vi "Juicer-ChangeMode.vi"(7 "Device reference":refnum<vi>, 8 "error in (no error)":errorcluster, 9 "Eventstring":string="auto-generate", 11 "Mode":enum16{"off", "reward", "flush", "purge"}(ring)) -> (0 "error out":errorcluster)   [LabVIEW 2015]
doc: "Changes the mode of a juicer device.\n\nDevice reference: what juicer?\nMode: what mode to switch to?\n off: All disconnected\n reward: Reward tank connected\n flush: Water flush tank connected\n purge: Pressurized air connected\nEventstring: used for timestamping\n--empty: no timestamp will be generated\n--unwired or \"auto-generate\": TS w/ default eventstring\n--otherwise: TS with user-provided string\n\nThe default eventstring is:\n[juicer name].changeMode.[mode]\n\nThis action involves multiple digital output writes; only the last one is timestamped."
uses:
  Typedefs/Juicer.ctl
  Rack/Typedefs/OutputRequest refnum.ctl
  Rack/Typedefs/OutputRequest.ctl
  Rack/Typedefs/InputData cluster.ctl
  Rack/Methods/Port drivers/DigitalInput-DataCluster.ctl
panel:
  # "(must be on same NI card)"
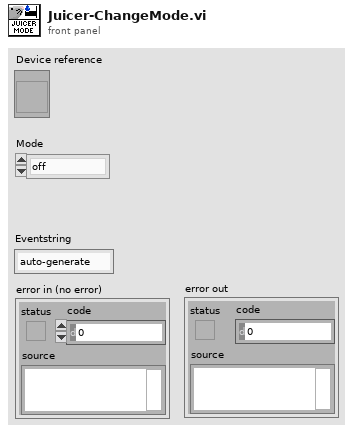
[diagram p1: front panel]
types:
  T1 = typedef "Juicer.ctl" = cluster{"Mode":enum16{"Off", "Juice/reward", "Water flush", "Air purge"}, "Settings":cluster{"Bleed #1 port index":i32, "Bleed #1 port name":string, "Bleed #2 port name":string, "Bleed #2 port index":i32, "Flush port name":string, "Flush port index":i32, "Purge port name":string, "Purge port index":i32, "Timestamp port name":string}, "OutputRequest event ref":T2, "InputData reference":refnum<vi>}
  T2 = typedef "OutputRequest refnum.ctl" = refnum<user-event>
  T3 = enum16{"Off", "Juice/reward", "Water flush", "Air purge"}
  T4 = typedef "OutputRequest.ctl" = cluster{"Target":string, "Command":string}
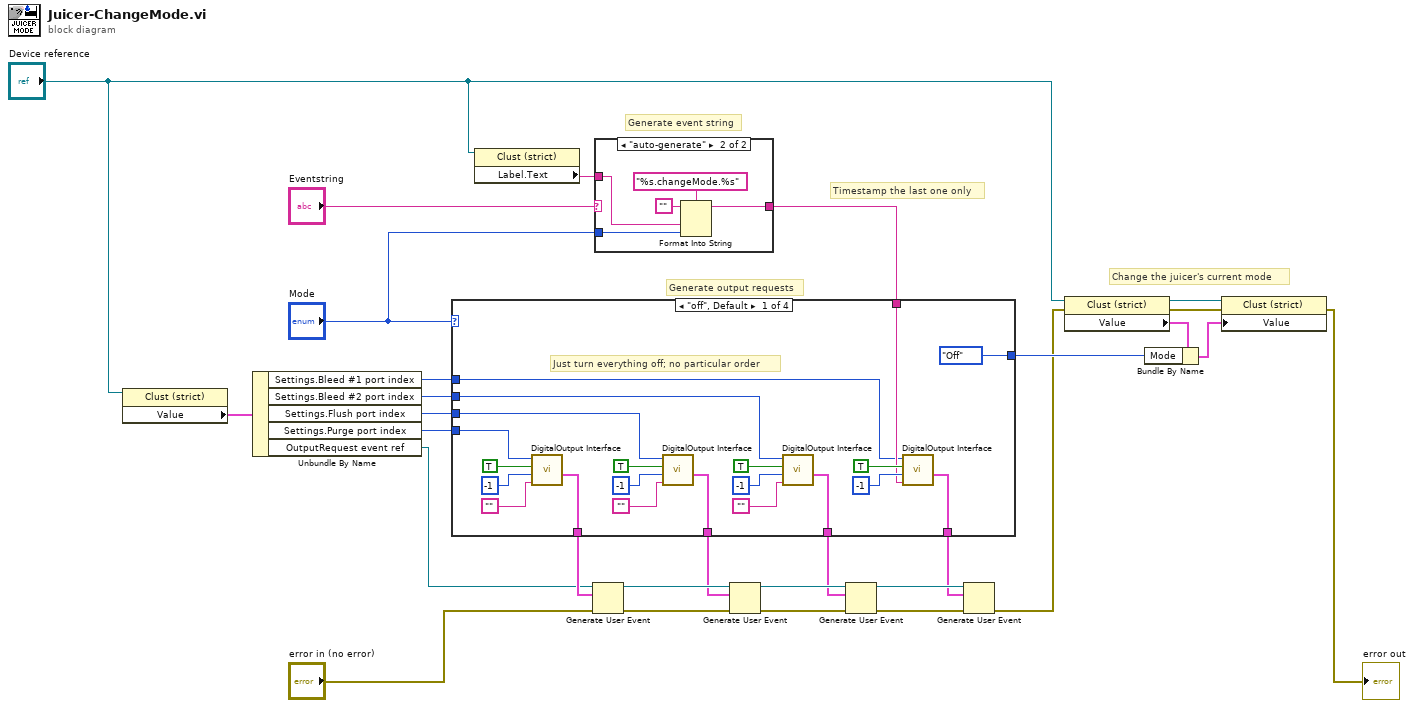
[diagram p0: block diagram]
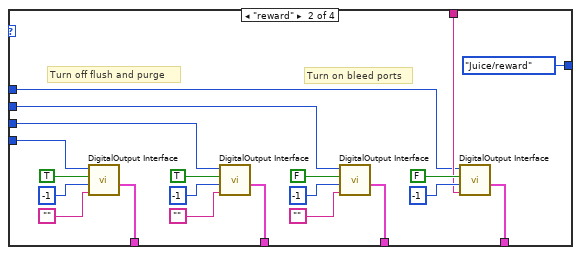
[diagram p2: hidden frame]
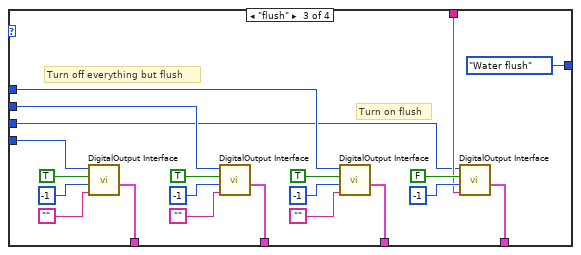
[diagram p3: hidden frame]
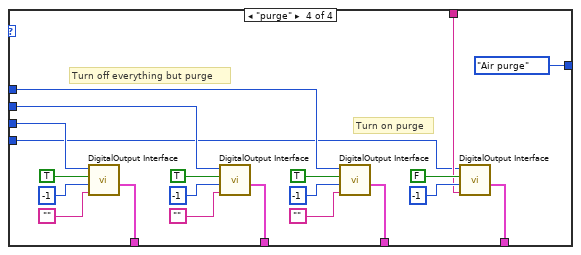
[diagram p4: hidden frame]
diagram:
  # "Change the juicer's current mode"
  # "Generate output requests"
  # "Timestamp the last one only"
  # "Generate event string"
  n1 = property class="Clust (strict)"(reference="Device reference") -> ("Value"=w29:T1)  [unwired: 1 in, 2 out]
  n2 = Unbundle By Name(w29) -> ("Settings.Bleed #1 port index"=w26:i32, "Settings.Bleed #2 port index"=w25:i32, "Settings.Flush port index"=w24:i32, "Settings.Purge port index"=w23:i32, "OutputRequest event ref"=w2:T2)
  n3 = property class="Clust (strict)"(reference="Device reference") -> ("Label.Text"=w27:string)  [unwired: 1 in, 2 out]
  n4 = case shown="\"auto-generate\"" "Eventstring" {
    selector: "Eventstring" -> [w30 _]
    tunnel: [w30 w33] -> w21
    tunnel: w27 -> [_ w32]
    tunnel: "Mode" -> [_ w31]
    frame Default {
      # "Use user-provided string"
    }
    frame "auto-generate" {
      n5 = Format Into String(format string="%s.changeMode.%s", initial string="", w32, w31) -> (resulting string=w33:string)  [unwired: 1 in, 1 out]
    }
  }
  n6 = case shown="\"off\", Default" "Mode" {
    tunnel: w26 -> [w40 w61 w80 w101]
    tunnel: w25 -> [w41 w62 w81 w102]
    tunnel: w24 -> [w42 w63 w79 w103]
    tunnel: w23 -> [w53 w74 w95 w100]
    tunnel: [w52 w73 w94 w116] -> w13
    tunnel: w21 -> [w43 w64 w85 w107]
    tunnel: [w39 w60 w84 w106] -> w12
    tunnel: [w38 w59 w83 w105] -> w11
    tunnel: [w37 w58 w82 w104] -> w10
    tunnel: [T3."Off" ("Mode") T3."Juice/reward" ("Mode") T3."Water flush" ("Mode") T3."Air purge" ("Mode")] -> w8
    frame "off", Default {
      # "Just turn everything off; no particular order"
      n7 = call "DigitalOutput Interface.vi"("Eventstring"="", "Pulse duration (-1 for cont.)"=-1, "On/off"=TRUE, "Port index"=w53) -> ("OutputRequest"=w52:T4)  [unwired: 7 in]
      n8 = call "DigitalOutput Interface.vi"("Eventstring"="", "Pulse duration (-1 for cont.)"=-1, "On/off"=TRUE, "Port index"=w42) -> ("OutputRequest"=w39:T4)  [unwired: 7 in]
      n9 = call "DigitalOutput Interface.vi"("Eventstring"="", "Pulse duration (-1 for cont.)"=-1, "On/off"=TRUE, "Port index"=w41) -> ("OutputRequest"=w38:T4)  [unwired: 7 in]
      n10 = call "DigitalOutput Interface.vi"("Eventstring"=w43, "Pulse duration (-1 for cont.)"=-1, "On/off"=TRUE, "Port index"=w40) -> ("OutputRequest"=w37:T4)  [unwired: 7 in]
    }
    frame "reward" {
      # "Turn on bleed ports"
      # "Turn off flush and purge"
      n11 = call "DigitalOutput Interface.vi"("Eventstring"="", "Pulse duration (-1 for cont.)"=-1, "On/off"=TRUE, "Port index"=w74) -> ("OutputRequest"=w73:T4)  [unwired: 7 in]
      n12 = call "DigitalOutput Interface.vi"("Eventstring"="", "Pulse duration (-1 for cont.)"=-1, "On/off"=TRUE, "Port index"=w63) -> ("OutputRequest"=w60:T4)  [unwired: 7 in]
      n13 = call "DigitalOutput Interface.vi"("Eventstring"="", "Pulse duration (-1 for cont.)"=-1, "On/off"=FALSE, "Port index"=w62) -> ("OutputRequest"=w59:T4)  [unwired: 7 in]
      n14 = call "DigitalOutput Interface.vi"("Eventstring"=w64, "Pulse duration (-1 for cont.)"=-1, "On/off"=FALSE, "Port index"=w61) -> ("OutputRequest"=w58:T4)  [unwired: 7 in]
    }
    frame "flush" {
      # "Turn on flush"
      # "Turn off everything but flush"
      n15 = call "DigitalOutput Interface.vi"("Eventstring"="", "Pulse duration (-1 for cont.)"=-1, "On/off"=TRUE, "Port index"=w95) -> ("OutputRequest"=w94:T4)  [unwired: 7 in]
      n16 = call "DigitalOutput Interface.vi"("Eventstring"="", "Pulse duration (-1 for cont.)"=-1, "On/off"=TRUE, "Port index"=w81) -> ("OutputRequest"=w84:T4)  [unwired: 7 in]
      n17 = call "DigitalOutput Interface.vi"("Eventstring"="", "Pulse duration (-1 for cont.)"=-1, "On/off"=TRUE, "Port index"=w80) -> ("OutputRequest"=w83:T4)  [unwired: 7 in]
      n18 = call "DigitalOutput Interface.vi"("Eventstring"=w85, "Pulse duration (-1 for cont.)"=-1, "On/off"=FALSE, "Port index"=w79) -> ("OutputRequest"=w82:T4)  [unwired: 7 in]
    }
    frame "purge" {
      # "Turn on purge"
      # "Turn off everything but purge"
      n19 = call "DigitalOutput Interface.vi"("Eventstring"="", "Pulse duration (-1 for cont.)"=-1, "On/off"=TRUE, "Port index"=w103) -> ("OutputRequest"=w116:T4)  [unwired: 7 in]
      n20 = call "DigitalOutput Interface.vi"("Eventstring"="", "Pulse duration (-1 for cont.)"=-1, "On/off"=TRUE, "Port index"=w102) -> ("OutputRequest"=w106:T4)  [unwired: 7 in]
      n21 = call "DigitalOutput Interface.vi"("Eventstring"="", "Pulse duration (-1 for cont.)"=-1, "On/off"=TRUE, "Port index"=w101) -> ("OutputRequest"=w105:T4)  [unwired: 7 in]
      n22 = call "DigitalOutput Interface.vi"("Eventstring"=w107, "Pulse duration (-1 for cont.)"=-1, "On/off"=FALSE, "Port index"=w100) -> ("OutputRequest"=w104:T4)  [unwired: 7 in]
    }
  }
  n23 = Generate User Event(user event=w2, event data cluster=w13, error in="error in (no error)") -> (user event out=w16:T2, error out=w19:errorcluster)  [unwired: 1 in]
  n24 = Generate User Event(user event=w16, event data cluster=w12, error in=w19) -> (user event out=w15:T2, error out=w18:errorcluster)  [unwired: 1 in]
  n25 = Generate User Event(user event=w15, event data cluster=w11, error in=w18) -> (user event out=w14:T2, error out=w17:errorcluster)  [unwired: 1 in]
  n26 = Generate User Event(user event=w14, event data cluster=w10, error in=w17) -> (error out=w5:errorcluster)  [unwired: 1 in, 1 out]
  n27 = property class="Clust (strict)"(reference="Device reference", error in=w5) -> (reference out=w6:refnum<vi>, error out=w1:errorcluster, "Value"=w9:T1)
  n28 = Bundle By Name(cluster=w9, "Mode"=w8) -> (w7:T1)
  n29 = property class="Clust (strict)"(reference=w6, error in=w1, "Value"=w7) -> (error out=→"error out":errorcluster)  [unwired: 1 out]
